vi "get ACS status.vi"(8 "error in (no error)":errorcluster, 11 "Channel in":refnum<class "Channel.lvclass">) -> (0 "error out":errorcluster, 3 "Channel out":refnum<class "Channel.lvclass">)   [LabVIEW 2018, in "Channel.lvclass"]
uses:
  Channel.lvclass
  Channel.lvclass/Channel.ctl
  RxTx/RxTx.lvclass
  Camera/Camera.lvclass
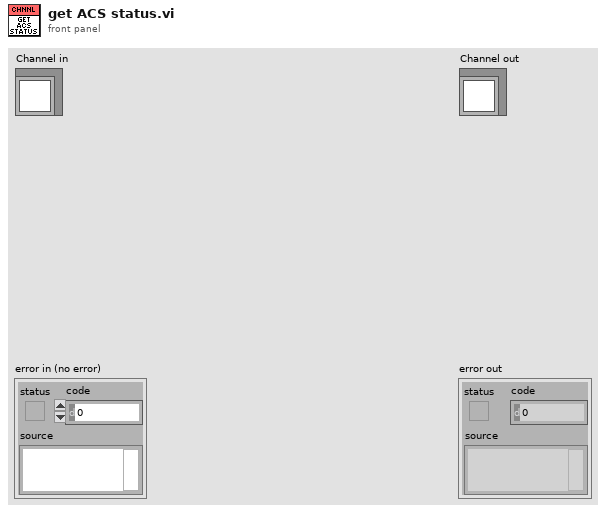
[diagram p1: front panel]
types:
  T1 = cluster{"CYCLES_DONE":u16, "LAST_IMAGE_NAME":string, "USED_DISK_SPACE":u16, "FRAMES_DONE":u16, "CCD_STATUS":string, "CURRENT_TEMPERATURE":i16, "TEMPERATURE_STATUS":string, "FRAME_EXPOSURE_TIME":sgl, "SERIAL_NUMBER":u16, "ACQUIRING":bool, "IMAGE_INDEX":u32, "POWER":bool, "ACS MODE":bool}
  T2 = cluster{"camera status":cluster{"CYCLES_DONE":u16, "LAST_IMAGE_NAME":string, "USED_DISK_SPACE":u16, "FRAMES_DONE":u16, "CCD_STATUS":string, "CURRENT_TEMPERATURE":i16, "TEMPERATURE_STATUS":string, "FRAME_EXPOSURE_TIME":sgl, "SERIAL_NUMBER":u16, "ACQUIRING":bool, "IMAGE_INDEX":u32, "POWER":bool, "ACS MODE":bool}}
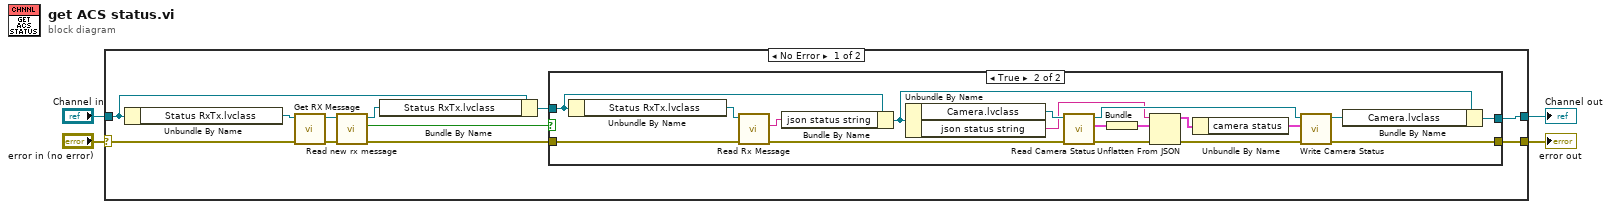
[diagram p0: block diagram]
diagram:
  n1 = case shown="No Error" "error in (no error)" {
    selector: "error in (no error)" -> [w12 w37]
    tunnel: [w15 w37] -> w3
    tunnel: [w14 w36] -> w1
    tunnel: "Channel in" -> [w7 w36]
    frame No Error {
      n2 = Unbundle By Name(w7) -> ("Status RxTx.lvclass"=w13:refnum<class "RxTx.lvclass">)
      n3 = call "Get RX Message.vi"("error in (no error)"=w12, "RxTx in"=w13) -> ("error out"=w11:errorcluster, "RxTx out"=w10:refnum<class "RxTx.lvclass">)  [unwired: 8 in]
      n4 = call-dynamic "Read new rx message.vi"("error in (no error)"=w11, "RxTx in"=w10) -> ("error out"=w8:errorcluster, "new rx message"=w9:bool, "RxTx out"=w6:refnum<class "RxTx.lvclass">)  [unwired: 7 in]
      n5 = Bundle By Name(cluster=w7, "Status RxTx.lvclass"=w6) -> (w5:refnum<class "Channel.lvclass">)
      n6 = case shown="True" w9 {
        tunnel: [w16 w25] -> w15
        tunnel: w5 -> [w17 w30]
        tunnel: [w17 w27] -> w14
        tunnel: w8 -> [w16 w32]
        frame False {
        }
        frame True {
          n7 = Unbundle By Name(w30) -> ("Status RxTx.lvclass"=w31:refnum<class "RxTx.lvclass">)
          n8 = call "Read Rx Message.vi"("error in (no error)"=w32, "RxTx in"=w31) -> ("error out"=w22:errorcluster, "Rx Message"=w23:string)  [unwired: 7 in, 1 out]
          n9 = Bundle By Name(cluster=w30, "json status string"=w23) -> (w28:refnum<class "Channel.lvclass">)
          n10 = Unbundle By Name(w28) -> ("Camera.lvclass"=w29:refnum<class "Camera.lvclass">, "json status string"=w26:string)
          n11 = call-dynamic "Read Camera Status.vi"("error in (no error)"=w22, "Camera in"=w29) -> ("error out"=w33:errorcluster, "camera status"=w21:T1, "Camera out"=w35:refnum<class "Camera.lvclass">)  [unwired: 7 in]
          n12 = Bundle("camera status"=w21) -> (w20:T2)  [unwired: 1 in]
          n13 = Unflatten From JSON(JSON string=w26, type and defaults=w20, error in (no error)=w33) -> (value=w19:T2, error out=w34:errorcluster)  [unwired: 4 in]
          n14 = Unbundle By Name(w19) -> ("camera status"=w18:T1)
          n15 = call-dynamic "Write Camera Status.vi"("error in (no error)"=w34, "Camera Status"=w18, "Camera in"=w35) -> ("error out"=w25:errorcluster, "Camera out"=w24:refnum<class "Camera.lvclass">)  [unwired: 7 in]
          n16 = Bundle By Name(cluster=w28, "Camera.lvclass"=w24) -> (w27:refnum<class "Channel.lvclass">)
        }
      }
    }
    frame Error {
    }
  }
  "error out" <- w3
  "Channel out" <- w1
